vi "getPixelArea.vi"(8 "error in (no error)":errorcluster, 10 "ReadOut Mode":dbl, 11 "WinX32Camera in":refnum<class "WinX32Camera.lvclass">) -> (0 "error out":errorcluster, 1 "yPixels":i32, 2 "xPixels":i32, 3 "WinX32Camera out":refnum<class "WinX32Camera.lvclass">)   [LabVIEW 2011, in "WinX32Camera.lvclass"]
uses:
  WinX32Camera.lvclass
  WinX32Camera.lvclass/WinX32Camera.ctl
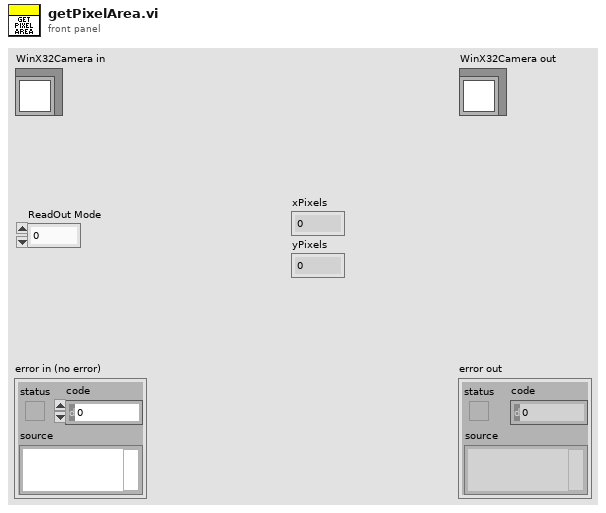
[diagram p1: front panel]
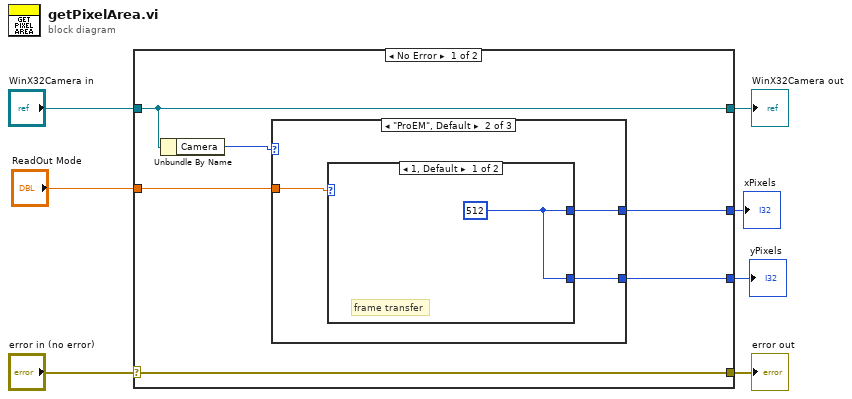
[diagram p0: block diagram]
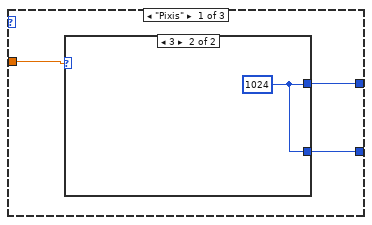
[diagram p2: hidden frame]
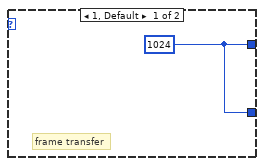
[diagram p3: hidden frame]
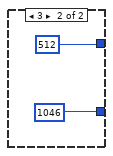
[diagram p4: hidden frame]
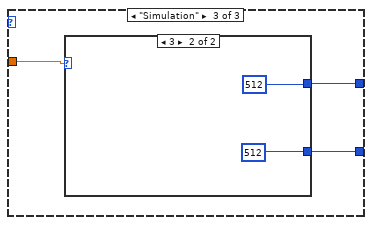
[diagram p5: hidden frame]
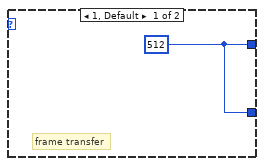
[diagram p6: hidden frame]
diagram:
  n1 = case shown="No Error" "error in (no error)" {
    selector: "error in (no error)" -> [w13 w32]
    tunnel: [w13 w32] -> w6
    tunnel: [w12 w31] -> w4
    tunnel: "WinX32Camera in" -> [w12 w31]
    tunnel: "ReadOut Mode" -> [w10 _]
    tunnel: [w9 _] -> w2
    tunnel: [w8 _] -> w1
    frame No Error {
      n2 = Unbundle By Name(w12) -> ("Camera"=w11:enum16{"Simulation", "Pixis", "ProEM"})
      n3 = case shown="\"ProEM\", Default" w11 {
        tunnel: w10 -> [w16 w21 w27]
        tunnel: [w15 w20 w26] -> w9
        tunnel: [w14 w19 w25] -> w8
        frame "Pixis" {
          n4 = case shown="3" w16 {
            tunnel: [w17 w18] -> w15
            tunnel: [w17 w18] -> w14
            frame 1, Default {
              w17 = 1024
              # "frame transfer"
            }
            frame 3 {
              w18 = 1024
            }
          }
        }
        frame "ProEM", Default {
          n5 = case shown="1, Default" w21 {
            tunnel: [w22 512] -> w20
            tunnel: [w22 1046] -> w19
            frame 1, Default {
              w22 = 512
              # "frame transfer"
            }
            frame 3 {
            }
          }
        }
        frame "Simulation" {
          n6 = case shown="3" w27 {
            tunnel: [w28 512] -> w26
            tunnel: [w28 512] -> w25
            frame 1, Default {
              w28 = 512
              # "frame transfer"
            }
            frame 3 {
            }
          }
        }
      }
    }
    frame Error {
    }
  }
  "error out" <- w6
  "WinX32Camera out" <- w4
  "xPixels" <- w2
  "yPixels" <- w1
